vi "Destroy.vi"(11 "Hello World Event in":refnum<class "Hello World Event.lvclass">) -> (3 "Hello World Event out":refnum<class "Hello World Event.lvclass">)   [LabVIEW 2021, in "Hello World Event.lvlib" / "Hello World Event.lvclass"]
uses:
  Hello World Event.lvclass
  Hello World Event.lvclass/Hello World Event.ctl
  jettl/jettl/Event jettl/Event jettl.lvclass
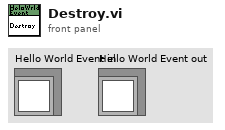
[diagram p1: front panel]
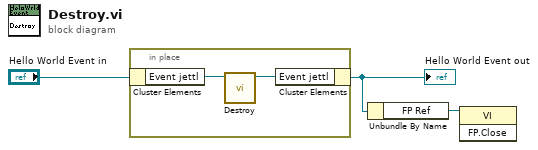
[diagram p0: block diagram]
diagram:
  n1 = in-place {
    n2 = in-place-cluster #1("Hello World Event in") -> ("Event jettl"=w5:refnum<class "Event jettl.lvclass">)
    n3 = call-dynamic "Destroy.vi"("jettl in"=w5) -> ("jettl out"=w4:refnum<class "Event jettl.lvclass">)  [unwired: 10 in]
    n4 = in-place-cluster #1("Event jettl"=w4) -> (w2:refnum<class "Hello World Event.lvclass">)
  }
  "Hello World Event out" <- w2
  n5 = Unbundle By Name(w2) -> ("FP Ref"=w3:refnum<vi>)
  n6 = invoke class="VI" method="FP.Close"(reference=w3) -> ()  [unwired: 2 in, 3 out]
